vi "PTScanner.contents.vi"   [LabVIEW 2014, in "PTScanner.lvlib"]
uses:
  PTScanner.lvlib
panel:
  # "Refer to block diagram for details"
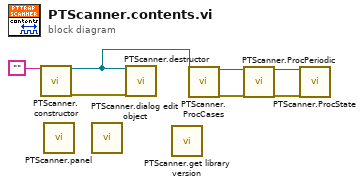
[diagram p0: block diagram]
diagram:
  n1 = call "PTScanner.constructor.vi"("name"="") -> ("i ref out"=w6:refnum<vi>, "error out"=w7:errorcluster)  [unwired: 16 in, 1 out]
  n2 = call "PTScanner.panel.vi"() -> ()  [unwired: 20 in]
  n3 = call "PTScanner.dialog edit object.vi"() -> ()  [unwired: 17 in, 3 out]
  n4 = call "PTScanner.destructor.vi"("i ref in"=w6, "error in (no error)"=w7) -> ()  [unwired: 17 in, 1 out]
  n5 = call "PTScanner.get library version.vi"() -> ()  [unwired: 1 in, 1 out]
  n6 = call "PTScanner.ProcCases.vi"("i ref in"=w6) -> ("i ref out"=w4:refnum<vi>, "error out"=w3:errorcluster)  [unwired: 16 in, 1 out]
  n7 = call "PTScanner.ProcPeriodic.vi"("i ref in"=w4, "error in (no error)"=w3) -> ("i ref out"=w2:refnum<vi>, "error out"=w1:errorcluster)  [unwired: 15 in, 1 out]
  n8 = call "PTScanner.ProcState.vi"("i ref in"=w2, "error in"=w1) -> ()  [unwired: 15 in, 3 out]
